vi "tm_waitnextframe.vi"(8 "error in (no error)":errorcluster {"code" format="%.0x"}, 10 "Timeout":i32=-1, 11 "Handle in":u32) -> (0 "error out":errorcluster {"code" format="%.0x"}, 1 "Frame Count":i32, 2 "Frame Index":i32, 3 "Handle out":u32)   [LabVIEW 2012]
uses:
  tmcamcon.dll
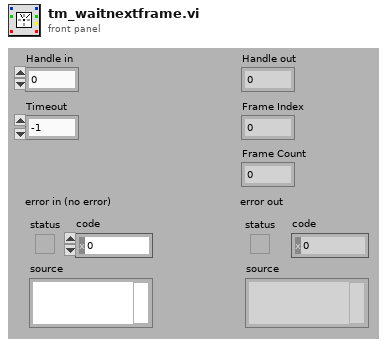
[diagram p1: front panel]
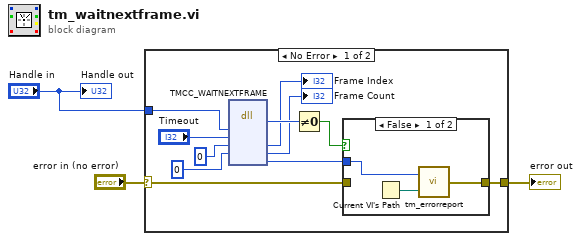
[diagram p0: block diagram]
diagram:
  n1 = case shown="No Error" "error in (no error)" {
    selector: "error in (no error)" -> [w7 w19]
    tunnel: [w4 w19] -> w2
    tunnel: "Handle in" -> [w12 _]
    frame No Error {
      n2 = dll-call lib="tmcamcon.dll" fn="TMCC_WAITNEXTFRAME"("HDCAM"=w12, "timeout"="Timeout", "frameindex"=0 ("Erval"), "framecount"=0 ("Erval")) -> ("return type"=w14:u32, "frameindex"=→"Frame Index":i32, "framecount"=→"Frame Count":i32, "Erval"=w6:i32)  [unwired: 6 in, 2 out]
      n3 = Not Equal To 0?(x=w14) -> (x != 0?=w5:bool)
      n4 = case shown="False" w5 {
        tunnel: w7 -> [_ w18]
        tunnel: [w16 w18] -> w4
        tunnel: w6 -> [w15 _]
        frame False {
          n5 = Current VI's Path() -> (path=w17:path)
          n6 = call "tm_errorreport.vi"("Source"=w17, "Error"=w15) -> ("error out"=w16:errorcluster)
        }
        frame True {
        }
      }
    }
    frame Error {
    }
  }
  "error out" <- w2
  "Handle out" <- "Handle in"
